vi "Koheras_get_set_Status.vi"(8 "error in":errorcluster, 9 "Answer-Length":i32[](array[numeric]), 10 "Command in":string[](array[string]), 11 "VISA resource name in":refnum<visa-resource-name>) -> (0 "error out":errorcluster, 2 "Return":string[](array[string]), 3 "VISA resource name out":refnum<visa-resource-name>)   [LabVIEW 2009]
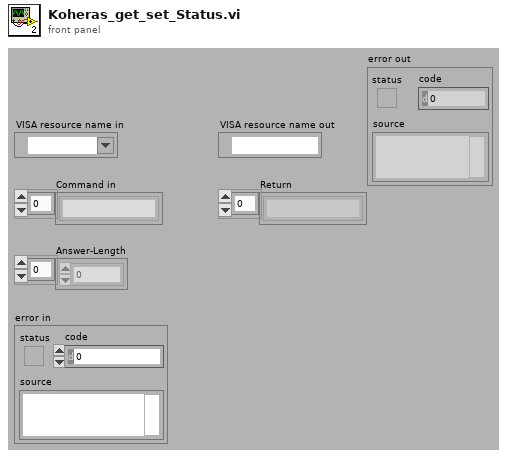
[diagram p1: front panel]
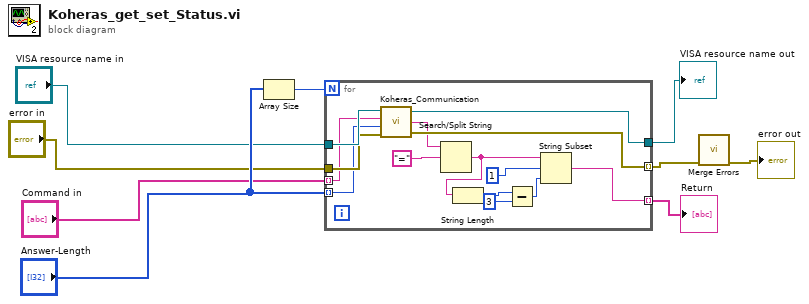
[diagram p0: block diagram]
diagram:
  n1 = Array Size(array="Answer-Length") -> (size(s)=w9:i32)
  n2 = for {
    N: w9 -> [_]
    tunnel: "VISA resource name in" -> [w23]
    tunnel: "error in" -> [w22]
    tunnel: [w21] -> w2 mode=indexing
    tunnel: [w20] -> w5
    tunnel: "Command in" -> [w19] mode=indexing
    tunnel: "Answer-Length" -> [w18] mode=indexing
    tunnel: [w15] -> w7 mode=indexing
    n3 = call "Koheras_Communication.vi"("Error in"=w22, "Answer length"=w18, "Command"=w19, "VISA resource name in"=w23) -> ("Error out"=w21:errorcluster, "Returns"=w17:string, "VISA resource name out"=w20:refnum<visa-resource-name>)
    n4 = Search/Split String(string=w17, search string/char (-)="=") -> (match + rest of string=w11:string)  [unwired: 3 out]
    n5 = String Length(string=w11) -> (length=w12:i32)
    n6 = Subtract(x=w12, y=3) -> (x-y=w14:i32)
    n7 = String Subset(string=w11, offset (0)=1, length (rest)=w14) -> (substring=w15:string)
  }
  "Return" <- w7
  "VISA resource name out" <- w5
  n8 = call <vilib>:"Merge Errors.vi"("error array in"=w2) -> ("error out"=→"error out":errorcluster)  [unwired: 3 in, 3 out]
